vi "Get Kasli Configuration.vi"(0 "Kasli in":refnum<class "Kasli.lvclass">=refnum, 5 "Kasli Name":string, 11 "error in (no error)":errorcluster) -> (3 "alias":string, 4 "Kasli out":refnum<class "Kasli.lvclass">, 6 "IP":string, 8 "ports":u32[](array[numeric]), 10 "repo":string, 14 "deviceDB":string, 15 "error out":errorcluster)   [LabVIEW 2020, in "CIRCUS_uServices.lvlib" / "Kasli Wrapper 2.0.lvlib" / "Kasli.lvclass"]
uses:
  Kasli.lvclass
  <vilib>/Utility/config.llb/NI_LVConfig.lvlib
  <vilib>/Utility/config.llb/Read Key (String).vi
  TALOS/TALOS_PPL.lvlibp
  <vilib>/Utility/config.llb/Read Key (U32).vi
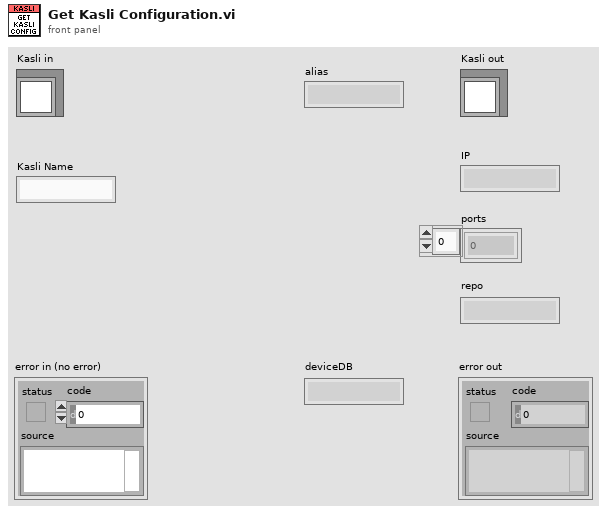
[diagram p1: front panel]
types:
  T1 = typedef "NI_LVConfig.lvlib/Config Data RefNum.ctl" = refnum<k1>
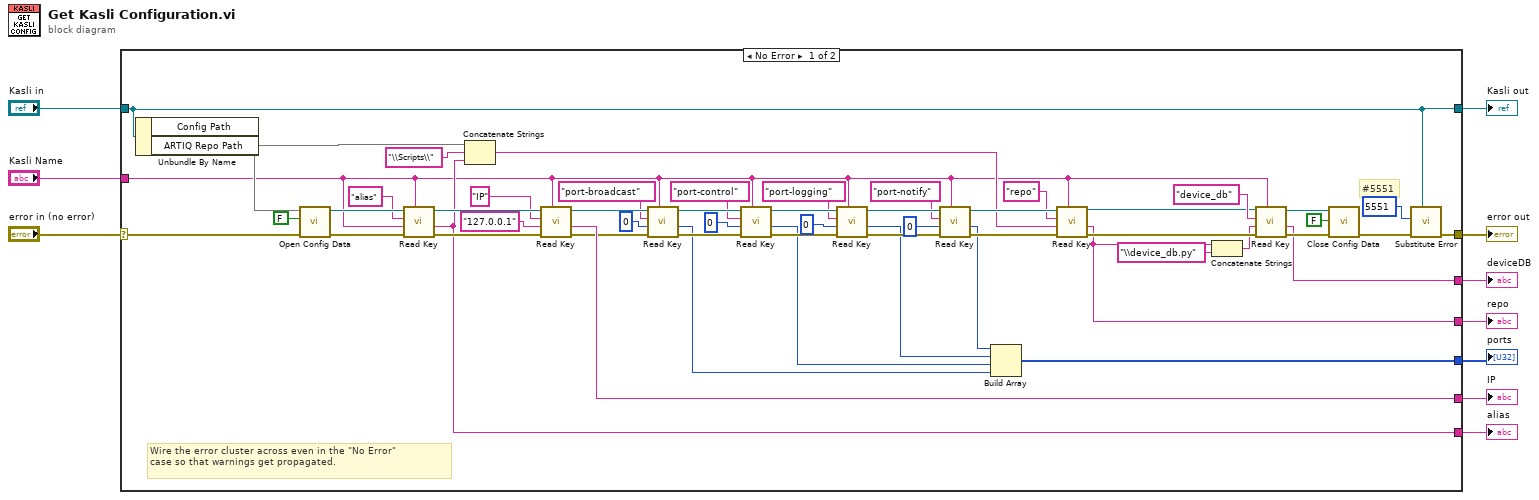
[diagram p0: block diagram]
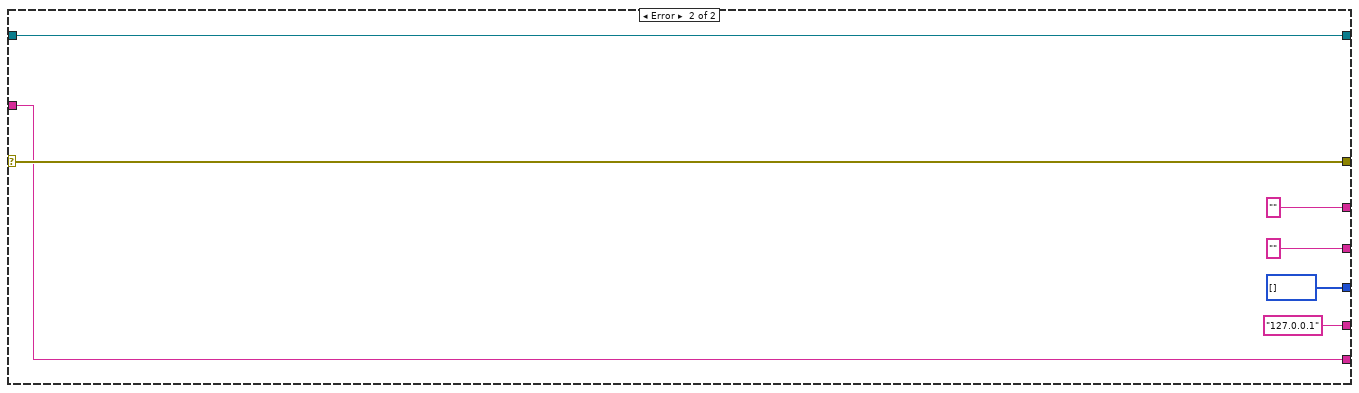
[diagram p2: hidden frame]
diagram:
  n1 = case shown="No Error" "error in (no error)" {
    selector: "error in (no error)" -> [w28 w71]
    tunnel: [w46 w71] -> w9
    tunnel: [w57 w70] -> w7
    tunnel: "Kasli in" -> [w57 w70]
    tunnel: "Kasli Name" -> [w17 w68]
    tunnel: [w22 w68] -> w5
    tunnel: [w44 "127.0.0.1" ("value")] -> w4
    tunnel: [w26 u32[] []] -> w3
    tunnel: [w15 "" ("value")] -> w2
    tunnel: [w12 "" ("value")] -> w1
    frame No Error {
      # "#5551"
      # "Wire the error cluster across even in the \"No Error\"\ncase so that warnings get propagated."
      n2 = Unbundle By Name(w57) -> ("Config Path"=w52, "ARTIQ Repo Path"=w24)
      n3 = call <vilib>:"Open Config Data.vi"("error in (no error)"=w28, "create file if necessary (T)"=FALSE, "configuration file path"=w52) -> ("error out"=w51:errorcluster, "refnum"=w56:T1)  [unwired: 6 in, 1 out]
      n4 = call-poly <vilib>:"Read Key.vi"("section"=w17, "error in (no error)"=w51, "default value"=w17, "key"="alias", "refnum"=w56) -> ("error out"=w54:errorcluster, "value"=w22:string, "refnum out"=w55:T1)  [unwired: 3 in, 1 out]
      n5 = Concatenate Strings(w24, "\\Scripts\\" ("string"), w22) -> (w21:string)
      n6 = call-poly <vilib>:"Read Key.vi"("section"=w17, "error in (no error)"=w54, "default value"="127.0.0.1", "key"="IP", "refnum"=w55) -> ("error out"=w29:errorcluster, "value"=w44:string, "refnum out"=w60:T1)  [unwired: 3 in, 1 out]
      n7 = call-poly <vilib>:"Read Key.vi"("section"=w17, "error in (no error)"=w29, "default value"=u32 0, "key"="port-broadcast", "refnum"=w60) -> ("error out"=w41:errorcluster, "value"=w30:u32, "refnum out"=w61:T1)  [unwired: 3 in, 1 out]
      n8 = call-poly <vilib>:"Read Key.vi"("section"=w17, "error in (no error)"=w41, "default value"=u32 0, "key"="port-control", "refnum"=w61) -> ("error out"=w36:errorcluster, "value"=w31:u32, "refnum out"=w62:T1)  [unwired: 3 in, 1 out]
      n9 = call-poly <vilib>:"Read Key.vi"("section"=w17, "error in (no error)"=w36, "default value"=u32 0, "key"="port-logging", "refnum"=w62) -> ("error out"=w59:errorcluster, "value"=w32:u32, "refnum out"=w63:T1)  [unwired: 3 in, 1 out]
      n10 = call-poly <vilib>:"Read Key.vi"("section"=w17, "error in (no error)"=w59, "default value"=u32 0, "key"="port-notify", "refnum"=w63) -> ("error out"=w58:errorcluster, "value"=w33:u32, "refnum out"=w64:T1)  [unwired: 3 in, 1 out]
      n11 = Build Array(w33, w32, w31, w30) -> (w26:u32[])
      n12 = call-poly <vilib>:"Read Key.vi"("section"=w17, "error in (no error)"=w58, "default value"=w21, "key"="repo", "refnum"=w64) -> ("error out"=w20:errorcluster, "value"=w15:string, "refnum out"=w11:T1)  [unwired: 3 in, 1 out]
      n13 = Concatenate Strings(w15, "\\device_db.py" ("string")) -> (w13:string)
      n14 = call-poly <vilib>:"Read Key.vi"("section"=w17, "error in (no error)"=w20, "default value"=w13, "key"="device_db", "refnum"=w11) -> ("error out"=w19:errorcluster, "value"=w12:string, "refnum out"=w18:T1)  [unwired: 3 in, 1 out]
      n15 = call <vilib>:"Close Config Data.vi"("error in (no error)"=w19, "write file if changed (T)"=FALSE, "refnum"=w18) -> ("error out"=w27:errorcluster)  [unwired: 7 in, 1 out]
      n16 = call "Substitute Error.vi"("LabVIEW Object"=w57, "error in (no error)"=w27, "Error Code"=5551) -> ("error out"=w46:errorcluster)  [unwired: 8 in]
    }
    frame Error {
    }
  }
  "error out" <- w9
  "Kasli out" <- w7
  "alias" <- w5
  "IP" <- w4
  "ports" <- w3
  "repo" <- w2
  "deviceDB" <- w1
